vi "Alarm.vi"   [LabVIEW 2017, in "Sefram DAS220.lvlib"]
doc: "Setup alarms to trig on a specific condition."
uses:
  <instrlib>/Sefram DAS220/Sefram DAS220.lvlib
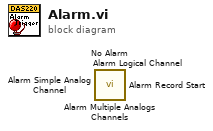
[diagram p0: block diagram]
diagram:
  n1 = call <instrlib>:"Alarm Multiple Analogs Channels.vi"() -> ()  [unwired: 10 in, 2 out]
  n2 = call <instrlib>:"Alarm Logical Channel.vi"() -> ()  [unwired: 10 in, 2 out]
  n3 = call <instrlib>:"Alarm Simple Analog Channel.vi"() -> ()  [unwired: 10 in, 2 out]
  n4 = call <instrlib>:"Alarm Record Start.vi"() -> ()  [unwired: 10 in, 2 out]
  n5 = call <instrlib>:"No Alarm.vi"() -> ()  [unwired: 10 in, 2 out]
